vi "Close TGM.vi"(8 "error in (no error)":errorcluster, 11 "Measurement Interface in":refnum<class "Measurement Interface.lvclass">) -> (0 "error out":errorcluster, 3 "Measurement Interface out":refnum<class "Measurement Interface.lvclass">)   [LabVIEW 2016, in "Measurement Interface.lvlib" / "Measurement Interface.lvclass"]
uses:
  Measurement Interface.lvclass
  Measurement Interface.lvclass/Measurement Interface.ctl
  Plugins/Test Group Manager.lvlibp/Test Group Manager.lvclass
  Test Group Manager/Read Test Group Manager.vi
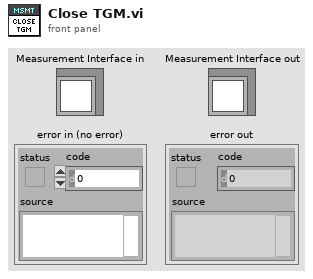
[diagram p1: front panel]
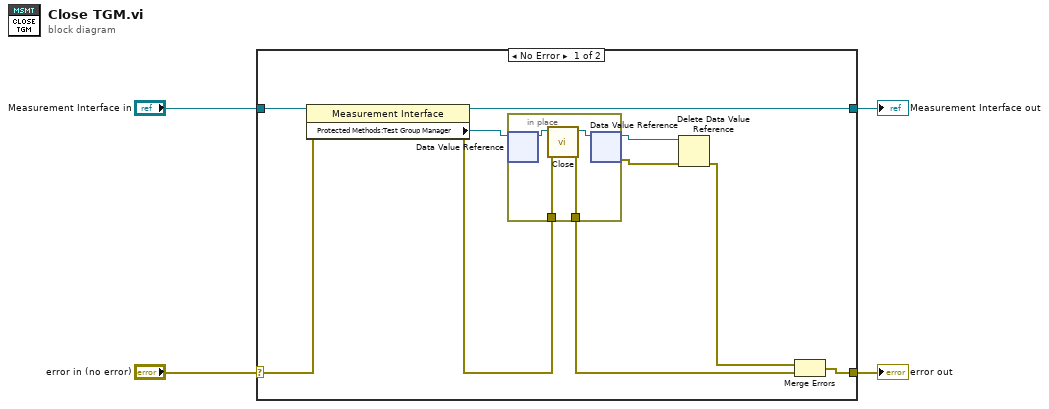
[diagram p0: block diagram]
diagram:
  n1 = case shown="No Error" "error in (no error)" {
    selector: "error in (no error)" -> [w14 w20]
    tunnel: [w6 w20] -> w3
    tunnel: [w12 w19] -> w1
    tunnel: "Measurement Interface in" -> [w13 w19]
    frame No Error {
      n2 = property class="Measurement Interface"(reference=w13, error in=w14) -> (reference out=w12:refnum<class "Measurement Interface.lvclass">, error out=w11:errorcluster, "Protected Methods:Test Group Manager"=w9:refnum<data-value>)
      n3 = in-place {
        in-place-border: w11 -> [w18]
        in-place-border: [w17] -> w10
        n4 = in-place-dvr #1(w9) -> (w16:refnum<class "Test Group Manager.lvclass">)  [unwired: 1 out]
        n5 = call "Close.vi"("error in (no error)"=w18, "Test Group Manager in"=w16) -> ("error out"=w17:errorcluster, "Test Group Manager out"=w15:refnum<class "Test Group Manager.lvclass">)  [unwired: 8 in]
        n6 = in-place-dvr #1(w15) -> (w8:refnum<data-value>, w7:errorcluster)
      }
      n7 = Delete Data Value Reference(data value reference=w8, error in=w7) -> (error out=w5:errorcluster)  [unwired: 1 out]
      n8 = Merge Errors(w5, w10) -> (w6:errorcluster)
    }
    frame Error {
    }
  }
  "error out" <- w3
  "Measurement Interface out" <- w1
